vi "HandleExit.vi"(8 "error in (no error)":errorcluster, 9 "VI Refnum":refnum<vi>, 10 "StopArgument":variant, 11 "ModuleAdmin":refnum<class "ModuleAdmin.lvclass">) -> (0 "error out":errorcluster, 1 "Exit via Stop Module Req?":bool, 2 "WaitForStop?":bool)   [LabVIEW 2014, in "FgenModule.lvlib"]
uses:
  FgenModule.lvlib
  <userlib>/NIST/ModuleAdminLib/ModuleAdmin/ModuleAdmin.lvclass
  PublicAPI/Arguments/Requests/clStopArgument.ctl
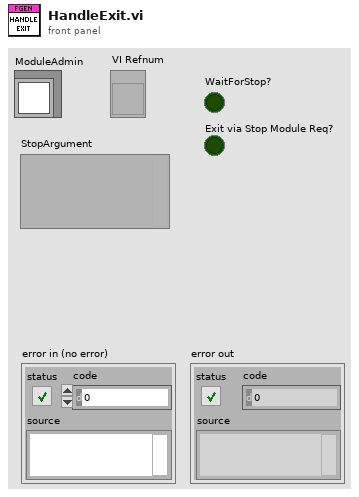
[diagram p1: front panel]
types:
  T1 = typedef "FgenModule.lvlib/clStopArgument.ctl" = cluster{"Exit via Stop Module Req?":bool, "Wait for Module to stop?":bool, "ModuleAdmin":refnum<class "ModuleAdmin.lvclass">}
  T2 = enum32{"Invalid", "Standard", "Closed", "Hidden", "Minimized", "Maximized"}
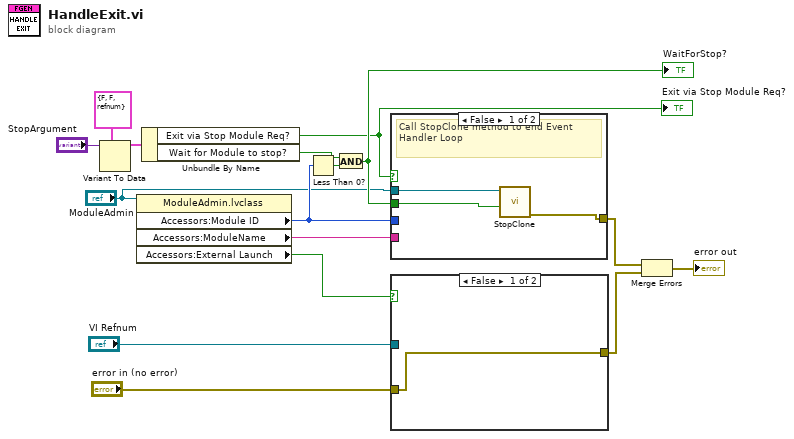
[diagram p0: block diagram]
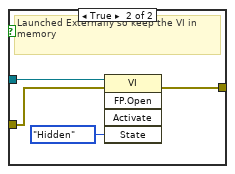
[diagram p2: hidden frame]
diagram:
  n1 = Variant To Data(type=T1 {"Exit via Stop Module Req?"=FALSE, "Wait for Module to stop?"=FALSE, "ModuleAdmin"=refnum} ("Stop Argument"), Variant="StopArgument") -> (data=w9:T1)  [unwired: 1 in, 1 out]
  n2 = property class="ModuleAdmin.lvclass"(reference="ModuleAdmin") -> ("Accessors:Module ID"=w4:i32, "Accessors:ModuleName"=w6:string, "Accessors:External Launch"=w7:bool)  [unwired: 1 in, 2 out]
  n3 = Unbundle By Name(w9) -> ("Exit via Stop Module Req?"=w2:bool, "Wait for Module to stop?"=w3:bool)
  "Exit via Stop Module Req?" <- w2
  n4 = Less Than 0?(x=w4) -> (x < 0?=w16:bool)
  n5 = And(x=w3, y=w16) -> (x .and. y?=w5:bool)
  "WaitForStop?" <- w5
  n6 = case shown="False" w2 {
    tunnel: w4 -> [_ _]
    tunnel: [w19 _] -> w13
    tunnel: w6 -> [_ _]
    tunnel: w5 -> [w18 _]
    tunnel: "ModuleAdmin" -> [w17 _]
    frame False {
      # "Call StopClone method to end Event Handler Loop"
      n7 = call "StopClone.vi"("Wait for Module to stop?"=w18, "ModuleAdmin"=w17) -> ("error out"=w19:errorcluster)  [unwired: 9 in]
    }
    frame True {
      # "This came from the Event Handler Loop"
    }
  }
  n8 = case shown="False" w7 {
    tunnel: "VI Refnum" -> [_ w24]
    tunnel: [w20 w22] -> w12
    tunnel: "error in (no error)" -> [w20 w21]
    frame False {
    }
    frame True {
      # "Launched Externally so keep the VI in memory"
      n9 = invoke class="VI" method="FP.Open"(reference=w24, error in=w21, "State"=T2."Hidden") -> (error out=w22:errorcluster)  [unwired: 2 in, 4 out]
    }
  }
  n10 = Merge Errors(w13, w12) -> (→"error out":errorcluster)
